vi "Plot Default Sine Cos Graph.vi"() -> ()   [LabVIEW 2020]
panel:
  out "Data":dbl[](array[numeric])
  out "Waveform Graph":dbl[][](graph)
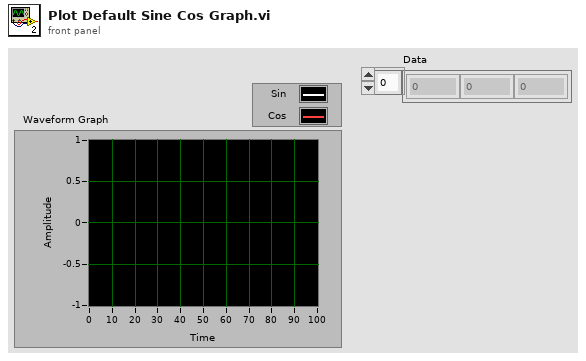
[diagram p1: front panel]
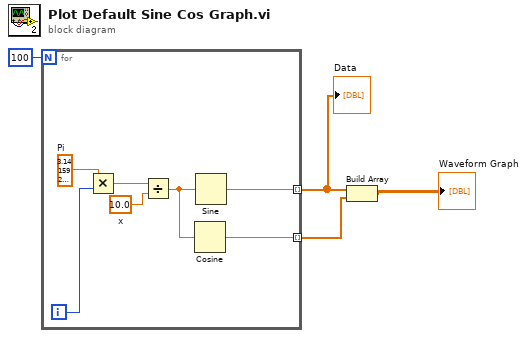
[diagram p0: block diagram]
diagram:
  n1 = for {
    N: 100 -> [_]
    tunnel: [w7] -> w3 mode=indexing
    tunnel: [w5] -> w2 mode=indexing
    i -> [w11]
    w8 = 10.0  # x
    w10 = 3.141592653589793  # Pi
    n2 = Multiply(x=w10, y=w11) -> (x*y=w9:dbl)
    n3 = Divide(x=w9, y=w8) -> (x/y=w6:dbl)
    n4 = Cosine(x=w6) -> (cos(x)=w5:dbl)
    n5 = Sine(x=w6) -> (sin(x)=w7:dbl)
  }
  "Data" <- w3
  n6 = Build Array(w3, w2) -> (→"Waveform Graph":dbl[][])
